vi "Multimeter_Init.vi"(8 "error in (no error)":errorcluster, 11 "MultimeterControl in":refnum<class "MultimeterControl.lvclass">) -> (0 "error out":errorcluster, 3 "MultimeterControl out":refnum<class "MultimeterControl.lvclass">)   [LabVIEW 2018, in "MultimeterControl.lvclass"]
uses:
  MultimeterControl.lvclass
  C:/Users/veral/Documents/itk-strip-sensor-qc/LabVIEW 2013/InstrControl/InstrControl.lvclass
  InstrControl.lvclass
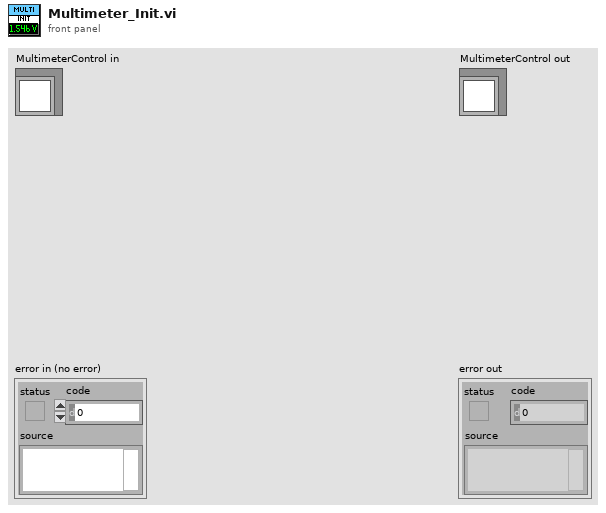
[diagram p1: front panel]
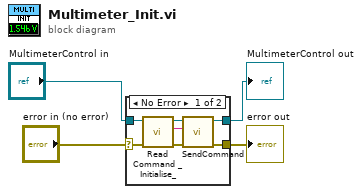
[diagram p0: block diagram]
diagram:
  n1 = case shown="No Error" "error in (no error)" {
    selector: "error in (no error)" -> [w8 w13]
    tunnel: [w10 w13] -> w3
    tunnel: [w11 w12] -> w1
    tunnel: "MultimeterControl in" -> [w9 w12]
    frame No Error {
      n2 = call-dynamic "Read Command _Initialise_.vi"("error in (no error)"=w8, "MultimeterControl in"=w9) -> ("error out"=w7:errorcluster, "Command \"Initialise\""=w6:string, "MultimeterControl out"=w5:refnum<class "MultimeterControl.lvclass">)  [unwired: 7 in]
      n3 = call "SendCommand.vi"("error in (no error)"=w7, "Command string"=w6, "InstControl in"=w5) -> ("error out"=w10:errorcluster, "InstControl out"=w11:refnum<class "MultimeterControl.lvclass">)  [unwired: 7 in]
    }
    frame Error {
    }
  }
  "error out" <- w3
  "MultimeterControl out" <- w1
